vi "Talon_SRX_limit_switch_just_read.vi"() -> ()   [LabVIEW 2020]
doc: "This example shows how to use a digital line to read a limit switch."
uses:
  <vilib>/Rock Robotics/WPI/ThirdParty/Phoenix-LabVIEW/Motor Controller/Controls/CTRE_Phoenix_MotorControl_ControlMode.ctl
  <vilib>/Rock Robotics/WPI/ThirdParty/Phoenix-LabVIEW/Motor Controller/Get/CTRE_Phoenix_MotorController_GetVoltage.vi
  <vilib>/Rock Robotics/WPI/ThirdParty/Phoenix-LabVIEW/Motor Controller/Get/CTRE_Phoenix_MotorController_GetLimitSwitchStates.vi
panel:
  out "Percent Output":dbl format="%16.4f"
  out "Forward Limit Closed?":bool
  out "Reverse Limit Closed?":bool
  in  "Motor\nOutput":dbl min=-1.0 max=1.0 step=0.01 format="%16.4f"
  in  "CAN Number":u8
  # "Set these inputs before running."
  # "roboRIO Wiring Diagram"
  # "Limit\nSwitch"
  # "COM"
  # "NC"
  # "NO"
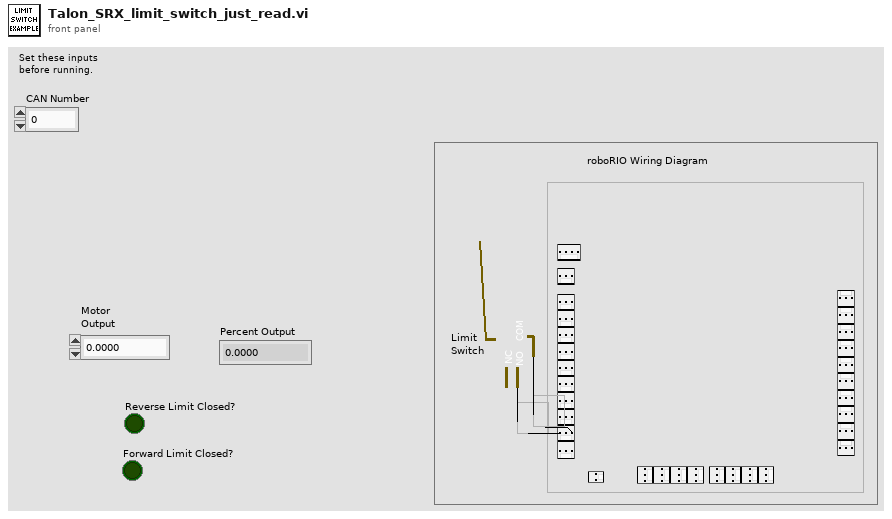
[diagram p1: front panel]
types:
  T1 = typedef "CTRE_Phoenix_MotorControl_ControlMode.ctl" = u16
  T2 = typedef "WPI_MotorControlDeviceRef.ctl" = cluster{"DeviceStatus":errorcluster, "Type":T3, "PWM":cluster{"PWM Channel":T4, "DeadBand":T5}, "CAN":cluster{"Device Number":u8, "SetOutput VI Ref":variant, "GetOutput VI Ref":variant, "Enable VI Ref":variant, "Disable VI Ref":variant, "Data":variant}, "Invert":bool, "DIO PWM":cluster{"PWM \"Enable\" Channel":T4, "DIOChannel":T6, "PWM Rate":dbl}}
  T3 = typedef "WPI_MotorControlType.ctl" = enum16{"PWM", "CAN", "DIO PWM"}
  T4 = typedef "FPGA_DIOPWMChannel.ctl" = enum8{"PWM 0", "PWM 1", "PWM 2", "PWM 3", "PWM 4", "PWM 5", "PWM 6", "PWM 7", "PWM 8", "PWM 9", "PWM MXP 0", "PWM MXP 1", "PWM MXP 2", "PWM MXP 3", "PWM MXP 4", "PWM MXP 5", "PWM MXP 6", "PWM MXP 7", "PWM MXP 8", "PWM MXP 9", "Invalid"}
  T5 = typedef "WPI_PWMDeadband.ctl" = cluster{"Name":string, "maxPositivePwm":i32, "minPositivePwm":i32, "centerPwm":i32, "maxNegativePwm":i32, "minNegativePwm":i32, "angularRange":u16}
  T6 = typedef "FPGA_DIOChannel.ctl" = enum8{"DIO 0", "DIO 1", "DIO 2", "DIO 3", "DIO 4", "DIO 5", "DIO 6", "DIO 7", "DIO 8", "DIO 9", "DIO MXP 0", "DIO MXP 1", "DIO MXP 2", "DIO MXP 3", "DIO MXP 4", "DIO MXP 5", "DIO MXP 6", "DIO MXP 7", "DIO MXP 8", "DIO MXP 9", "DIO MXP 10", "DIO MXP 11", "DIO MXP 12", "DIO MXP 13", "DIO MXP 14", "DIO MXP 15", "SPI Port CS1", "SPI Port CS2", "SPI Port CS3", "SPI Port MISO", "SPI Port MOSI", "Invalid"}
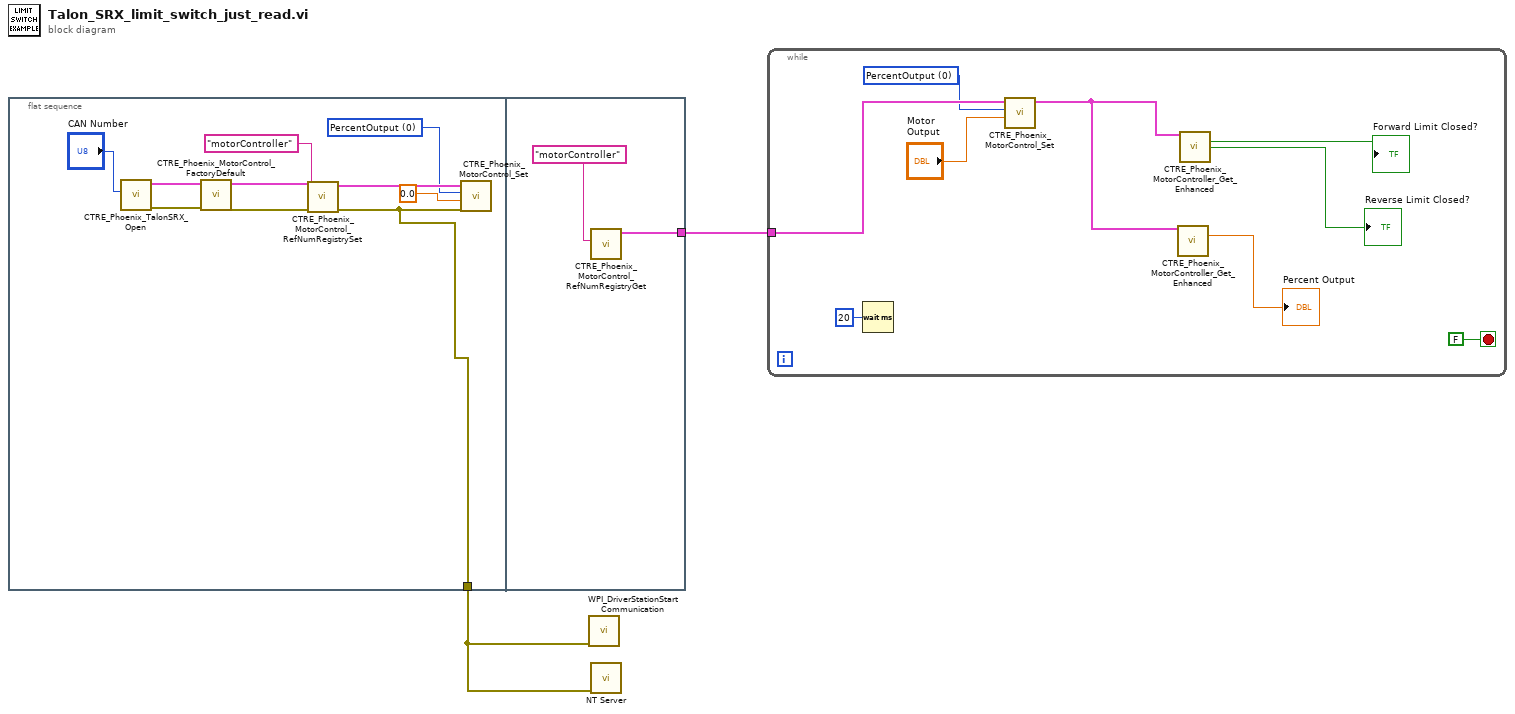
[diagram p0: block diagram]
diagram:
  n1 = flat-sequence {
    tunnel: [w5] -> w1
    tunnel: [w13] -> w2
    frame #0 {
      w10 = T1 0 items=["PercentOutput"=0, "Position"=1, "Velocity"=2, "Current"=3, "Follower"=5, "MotionProfile"=6, "MotionMagic"=7, "MotionMagicArc"=8, "MotionProfileArc"=10, "Disabled"=15] ("Control Mode")
      n2 = call <vilib>:"CTRE_Phoenix_TalonSRX_Open.vi"("Device Number"="CAN Number") -> ("error out"=w8:errorcluster, "PhoenixMotorControlDevRef"=w7:T2)  [unwired: 9 in]
      n3 = call <vilib>:"CTRE_Phoenix_MotorControl_FactoryDefault.vi"("error in"=w8, "PhoenixMotorControlDevRef"=w7) -> ("error out"=w3:errorcluster, "PhoenixMotorControlDevRef"=w4:T2)  [unwired: 8 in]
      n4 = call <vilib>:"CTRE_Phoenix_MotorControl_RefNumRegistrySet.vi"("error in (no error)"=w3, "refnum name"="motorController", "PhoenixMotorControlDevRef"=w4) -> ("error out"=w5:errorcluster, "PhoenixMotorControlDevRef"=w11:T2)  [unwired: 7 in]
      n5 = call <vilib>:"CTRE_Phoenix_MotorControl_Set.vi"("error in (no error)"=w5, "Output"=0.0, "Control Mode"=w10, "PhoenixMotorControlDevRef"=w11) -> ()  [unwired: 6 in, 2 out]
    }
    frame #1 {
      n6 = call <vilib>:"CTRE_Phoenix_MotorControl_RefNumRegistryGet.vi"("refnum name"="motorController") -> ("PhoenixMotorControlDevRef"=w13:T2)  [unwired: 9 in, 1 out]
    }
  }
  n7 = call <vilib>:"WPI_DriverStationStart Communication.vi"("error in (no error)"=w1) -> ()  [unwired: 11 in]
  n8 = call <vilib>:"NT Server.vi"("error in (no error)"=w1) -> ()  [unwired: 11 in]
  n9 = while {
    tunnel: w2 -> [w21]
    stop <- FALSE stop-if-true
    w20 = T1 0 items=["PercentOutput"=0, "Position"=1, "Velocity"=2, "Current"=3, "Follower"=5, "MotionProfile"=6, "MotionMagic"=7, "MotionProfileArc"=10, "Disabled"=15] ("Control Mode")
    n10 = Wait (ms)(milliseconds to wait=u32 20) -> ()  [unwired: 1 out]
    n11 = call <vilib>:"CTRE_Phoenix_MotorControl_Set.vi"("Output"="Motor\nOutput", "Control Mode"=w20, "PhoenixMotorControlDevRef"=w21) -> ("PhoenixMotorControlDevRef"=w16:T2)  [unwired: 7 in, 1 out]
    n12 = call-poly <vilib>:"CTRE_Phoenix_MotorController_Get_Enhanced.vi"("PhoenixMotorControlDevRef"=w16) -> ("Percent Output"=→"Percent Output":dbl)  [unwired: 10 in, 4 out]
    n13 = call-poly <vilib>:"CTRE_Phoenix_MotorController_Get_Enhanced.vi"("PhoenixMotorControlDevRef"=w16) -> ("Forward Limit Closed?"=→"Forward Limit Closed?":bool, "Reverse Limit Closed?"=→"Reverse Limit Closed?":bool)  [unwired: 11 in, 2 out]
  }
